vi "Create-value-reference.vi"(8 "error in (no error)":errorcluster) -> (0 "error out":errorcluster, 3 "UI ref.":refnum<data-value>)   [LabVIEW 2013, in "CameraVision.lvlib" / "CV-UI.lvclass"]
uses:
  CV-UI.lvclass
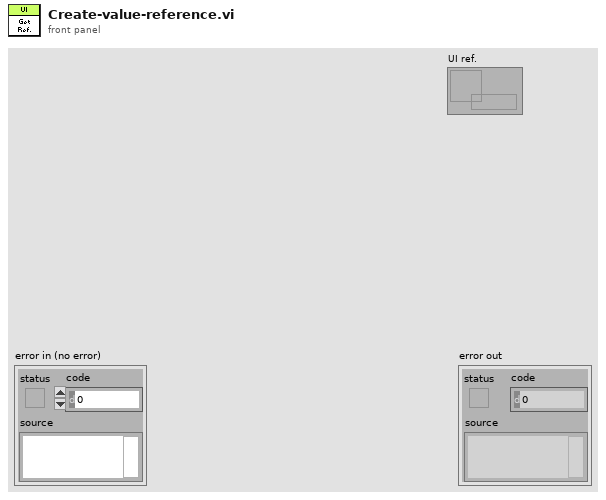
[diagram p1: front panel]
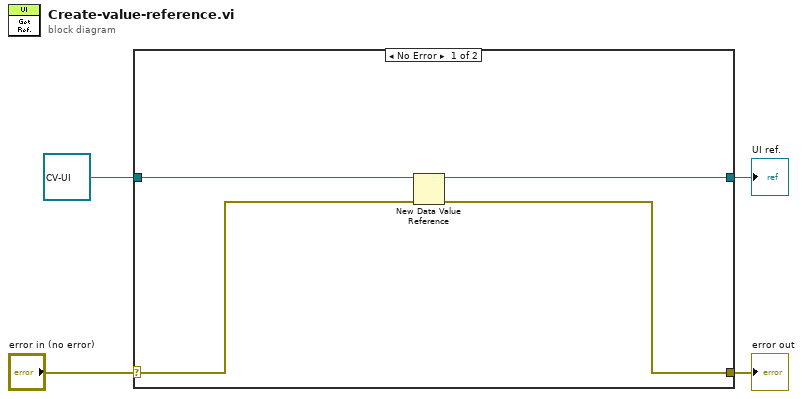
[diagram p0: block diagram]
diagram:
  n1 = case shown="No Error" "error in (no error)" {
    selector: "error in (no error)" -> [w7 w9]
    tunnel: [w6 w9] -> w3
    tunnel: refnum<class "CV-UI.lvclass"> refnum ("UI in") -> [w5 _]
    tunnel: [w8 _] -> w1
    frame No Error {
      n2 = New Data Value Reference(data value=w5, error in=w7) -> (data value reference=w8:refnum<data-value>, error out=w6:errorcluster)
    }
    frame Error {
    }
  }
  "error out" <- w3
  "UI ref." <- w1
